vi "CRC_add.vi"(8 "error in (no error)":errorcluster, 11 "Felica DOWN in":refnum<class "Felica DOWN.lvclass">) -> (0 "error out":errorcluster, 3 "Felica DOWN out":refnum<class "Felica DOWN.lvclass">)   [LabVIEW 2019, in "Felica DOWN.lvclass"]
uses:
  Felica DOWN.lvclass
  TypeDef/Store.ctl
  Felica DOWN.lvclass/Felica DOWN.ctl
  Libraries/CRC/CRC16CITT_A_F.vi
  RFID system.lvclass
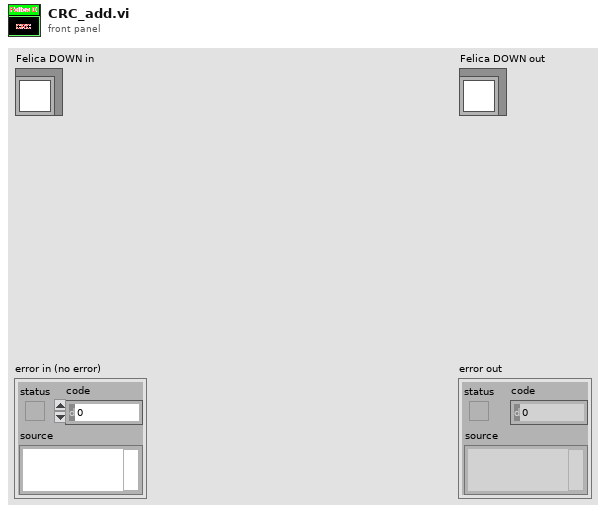
[diagram p1: front panel]
types:
  T1 = typedef "Store.ctl" = enum16{"envelope", "noise", "demSubCar", "CH_frame", "Decode", "demodulate", "in", "out", "sum", "subCarrier", "frame", "command", "encode", "modulate", "encode_UP", "modulate_up", "demod_up", "envelop_up", "sum_up", "out_up", "in_up"}
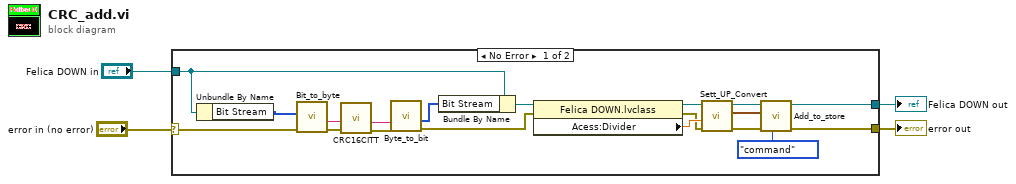
[diagram p0: block diagram]
diagram:
  n1 = case shown="No Error" "error in (no error)" {
    selector: "error in (no error)" -> [w22 w24]
    tunnel: [w14 w24] -> w3
    tunnel: "Felica DOWN in" -> [w21 w25]
    tunnel: [w16 w25] -> w1
    frame No Error {
      n2 = Unbundle By Name(w21) -> ("Bit Stream"=w23:u8[])
      n3 = call "Bit_to_byte.vi"("Error In"=w22, "Array of bit"=w23) -> ("Error Out"=w11:errorcluster, "BYTE"=w12:string)  [unwired: 7 in, 1 out]
      n4 = call-poly "CRC16CITT.vi"("Error In"=w11, "DATA PACKET"=w12) -> ("Error Out"=w10:errorcluster, "DATA PACKET+CRC"=w9:string)  [unwired: 7 in, 1 out]
      n5 = call "Byte_to_bit.vi"("Error In"=w10, "BYTE"=w9) -> ("Error Out"=w6:errorcluster, "Arrray of bit (str)"=w20:u8[])  [unwired: 5 in, 1 out]
      n6 = Bundle By Name(cluster=w21, "Bit Stream"=w20) -> (w19:refnum<class "Felica DOWN.lvclass">)
      n7 = property class="Felica DOWN.lvclass"(reference=w19, error in=w6) -> (reference out=w8:refnum<class "Felica DOWN.lvclass">, error out=w5:errorcluster, "Acess:Divider"=w7:dbl)
      n8 = call-dynamic "Sett_UP_Convert.vi"("error in (no error)"=w5, "Divider(1)"=w7, "Felica DOWN in"=w8) -> ("error out"=w15:errorcluster, "Waveform"=w18:waveform(dbl), "Felica DOWN out"=w17:refnum<class "Felica DOWN.lvclass">)  [unwired: 6 in]
      n9 = call "Add_to_store.vi"("Store"=Store."command", "error in (no error)"=w15, "Waveform"=w18, "RFID system in"=w17) -> ("error out"=w14:errorcluster, "RFID system out"=w16:refnum<class "Felica DOWN.lvclass">)  [unwired: 6 in]
    }
    frame Error {
    }
  }
  "error out" <- w3
  "Felica DOWN out" <- w1
